vi "XY Graph Get Plot Metadata Type.vi"(8 "Error In":errorcluster, 11 "Graph Label":string) -> (0 "Error Out":errorcluster, 1 "Found?":bool, 3 "Plot Metadata Type":variant)   [LabVIEW 2019, in "XY Graph Add-Ons.lvlib"]
uses:
  XY Graph Add-Ons.lvlib
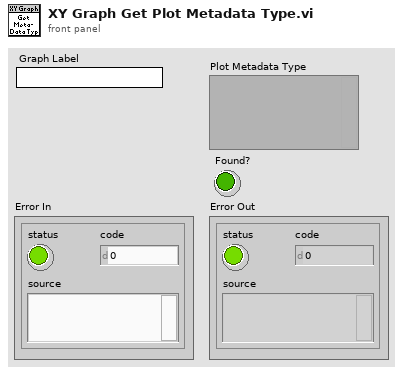
[diagram p1: front panel]
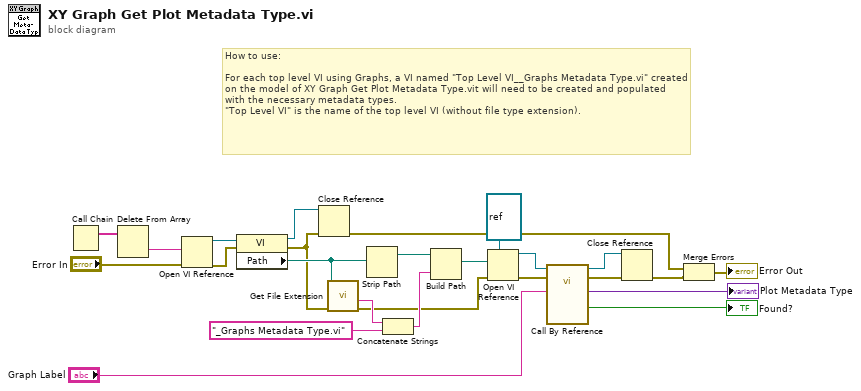
[diagram p0: block diagram]
diagram:
  # "How to use:\n\nFor each top level VI using Graphs, a VI named \"Top Level VI__Graphs Metadata Type.vi\" created on the model of XY Graph Get Plot Metadata Type.vit will need to be created and populated with the necessary metadata types.\n\"Top Level VI\" is the name of the top level VI (without file type extension)."
  n1 = Call Chain() -> (call chain=w25:string[])
  n2 = Delete From Array(array=w25) -> (deleted portion=w19:string)  [unwired: 2 in, 1 out]
  n3 = Open VI Reference(vi path=w19, error in (no error)="Error In") -> (vi reference=w23:refnum<vi>, error out=w22:errorcluster)  [unwired: 4 in]
  n4 = property class="VI"(reference=w23, error in=w22) -> (reference out=w17:refnum<vi>, error out=w9:errorcluster, "Path"=w18:path)
  n5 = Close Reference(reference=w17, error in (no error)=w9) -> (error out=w2:errorcluster)
  n6 = call <vilib>:"Get File Extension.vi"("error in (no error)"=w9, "file"=w18) -> ("error out"=w13:errorcluster, "filename without extension"=w16:string)  [unwired: 5 in, 3 out]
  n7 = Strip Path(path=w18) -> (stripped path=w21:path)  [unwired: 1 out]
  n8 = Concatenate Strings(w16, "_Graphs Metadata Type.vi" ("string")) -> (w15:string)
  n9 = Build Path(base path=w21, name or relative path=w15) -> (appended path=w14:path)
  n10 = Open VI Reference(type specifier VI Refnum (for type only)=refnum<vi> refnum, vi path=w14, error in (no error)=w13) -> (vi reference=w7:refnum<vi>, error out=w8:errorcluster)  [unwired: 3 in]
  n11 = call-by-ref "?"(reference=w7, error in=w8, "Graph Label"="Graph Label") -> (reference out=w5:refnum<vi>, error out=w4:errorcluster, "Found?"=→"Found?":bool, "Plot Metadata Type"=→"Plot Metadata Type":variant)  [unwired: 9 in]
  n12 = Close Reference(reference=w5, error in (no error)=w4) -> (error out=w3:errorcluster)
  n13 = Merge Errors(w2, w3) -> (→"Error Out":errorcluster)
